vi "WiFi HttpUpload_Camera.vi"   [LabVIEW 2014]
doc: "This example shows how to take a picuture from ArduCAM mini 2MP camera and upload to HTTP server."
uses:
  PWS_ESP8266/PWS_ESP8266.lvlib
  QwaveSys_Interface/QwaveSys_Interface.lvlib
panel:
  # "Overview: Demonstrates how to use  HTTP upload function with AduCAM 2MP API to upload JPEG image to server. *ArduCAM required both SPI and I2C interface. (*I2C is for communication with PWS and SPI is for transfer image from FIFO buffer at high speed)\nRequirements: LabVIEW Full Development System,Arduino Compatible Compiler for LabVIEW,Programmable Wireless Stamp (PWS) Library.\nInstructions:\n1. Wire the ArduCAM to the Pmod SPI interface. refer below diagram.\n2. Wire the SCL,SDA from ArduCAM to the  I2C connector. refer below diagram. \n3. If this example has been loaded from the Arduino Compatible Compiler for LabVIEW, simply select Compile and Download.  Otherwise, open Tools>Arduino Compatible Compiler for LabVIEW in LabVIEW, then select File>Load VI, and select this VI and then Compile and Download.\n4. Open \"Serial Monitor\" by select \"Tools>Serial Monitor\" and select baud rate to 9600.\n5. Observe the data being print out on serial port monitor and RED led at USB TX LED will be blinking, by default at serial monitor it's will shown \"Event Connecting: (6) WL_DISCONNECTED\"\n6. Press and Hold FPROM_Btn for 2 sec or more to enter Smart Config mode. At serial monitor window its will shown \"Smart_Config_enter\"\n7. Using Smart Config Apps on Andriod/iOS to configure the WiFi network. refer getting start document for more information.\n8. After PWS has configured wifi network successfully. Observe  the \"Image Size: \" data being print out on serial port monitor. \n9. Goto \"http://iosys.link/pws/uploads/test.jpg\" to view the uploaded image file.\n\n#NOTE: \nArduCAM mini 2MP. The Arduino compatible based camera is a 2MP pixel camera sensor that supports output for raw RGB, RGB556/555, GRB422, YUV (422/420), YCbCr (4:2:2) and JPEG compression formats. This sensor is a great option for real time simple video applications.\nRefer: http://www.arducam.com/arducam-mini-released/"
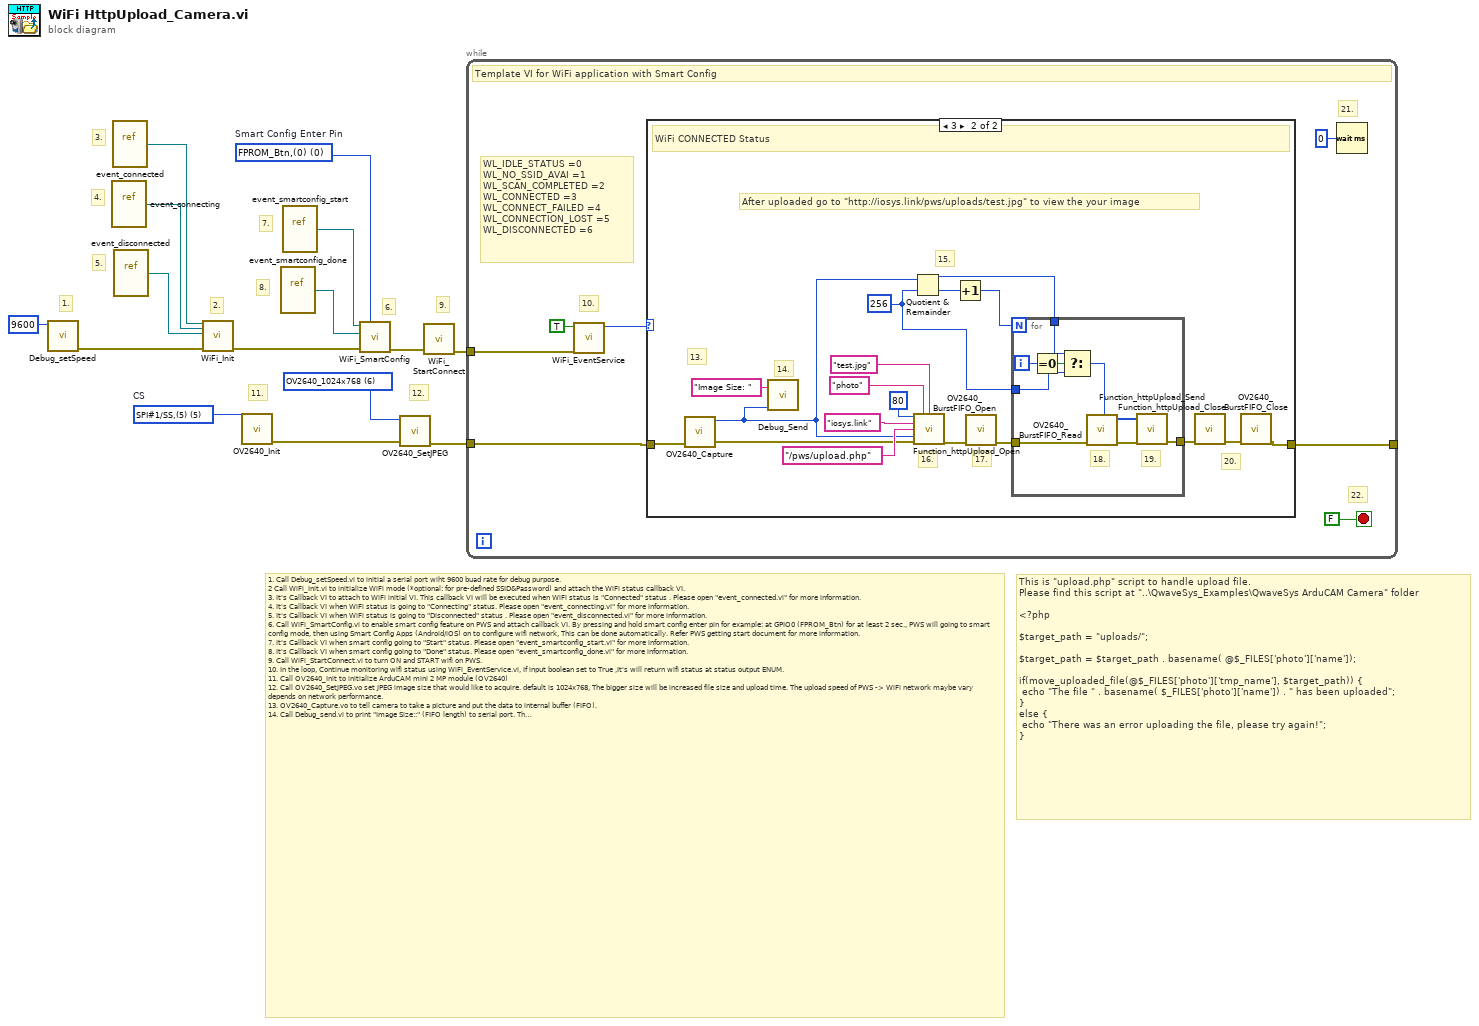
[diagram p0: block diagram]
diagram:
  w2 = u8 5 items=["SPI#1/SS,(5)"=5, "SPI#2/MOSI,(13)"=13, "SPI#3/MISO,(12)"=12, "SPI#4/SCLK,(14)"=14, "UART#1/CS,(15)"=15, "UART#2/TXD,(1)"=1, "UART#3/RXD,(3)"=3, "UART#4/LED,(16)"=16, "FPROM_Btn,(0)"=0, "SDCard_CS,(4)"=4, "I2C-SDA/TXD1,(2)"=2, "ADC0,(17)"=17]  # CS
  w4 = u16 6 items=["OV2640_160x120", "OV2640_176x144", "OV2640_320x240", "OV2640_352x288", "OV2640_640x480", "OV2640_800x600", "OV2640_1024x768", "OV2640_1280x1024", "OV2640_1600x1200"] ("resolution")
  w8 = u8 0 items=["SPI#1/SS,(5)"=5, "SPI#2/MOSI,(13)"=13, "SPI#3/MISO,(12)"=12, "SPI#4/SCLK,(14)"=14, "UART#1/CS,(15)"=15, "UART#2/TXD,(1)"=1, "UART#3/RXD,(3)"=3, "UART#4/LED,(16)"=16, "FPROM_Btn,(0)"=0, "SDCard_CS,(4)"=4, "I2C-SDA/TXD1,(2)"=2, "ADC0,(17)"=17]  # Smart Config Enter Pin
  # "This is \"upload.php\" script to handle upload file. \nPlease find this script at \"..\\QwaveSys_Examples\\QwaveSys ArduCAM Camera\" folder \n\n<?php\n\n$target_path = \"uploads/\";\n\n$target_path = $target_path . basename( @$_FILES['photo']['name']);\n\nif(move_uploaded_file(@$_FILES['photo']['tmp_name'], $target_path)) {\n\techo \"The file \" . basename( $_FILES['photo']['name']) . \" has been uploaded\";\n}\nelse {\n\techo \"There was an error uploading the file, please try again!\";\n}"
  # "12."
  # "11."
  # "9."
  # "8."
  # "7."
  # "1. Call Debug_setSpeed.vi to initial a serial port wiht 9600 buad rate for debug purpose.\n2 Call WiFi_Init.vi to initialize WiFi mode (*optional: for pre-defined SSID&Password) and attach the WiFi status callback VI.\n3. It's Callback VI to attach to WiFi initial VI. This callback VI will be executed when WiFi status is \"Connected\" status . Please open \"event_connected.vi\" for more information.\n4. It's Callback VI when WiFi status is going to \"Connecting\" status. Please open \"event_connecting.vi\" for more information.\n5. It's Callback VI when WiFi status is going to \"Disconnected\" status . Please open \"event_disconnected.vi\" for more information.\n6. Call WiFi_SmartConfig.vi to enable smart config feature on PWS and attach callback VI. By pressing and hold smart config enter pin for example: at GPIO0 (FPROM_Btn) for at least 2 sec., PWS will going to smart config mode, then using Smart Config Apps (Android/iOS) on to configure wifi network, This can be done automatically. Refer PWS getting start document for more information.\n7. It's Callback VI when smart config going to \"Start\" status. Please open \"event_smartconfig_start.vi\" for more information.\n8. It's Callback VI when smart config going to \"Done\" status. Please open \"event_smartconfig_done.vi\" for more information.\n9. Call WiFi_StartConnect.vi to turn ON and START wifi on PWS.\n10. In the loop, Continue monitoring wifi status using WiFi_EventService.vi, If input boolean set to True ,It's will return wifi status at status output ENUM. \n11. Call OV2640_Init to initialize ArduCAM mini 2 MP module (OV2640)\n12. Call OV2640_SetJPEG.vo set JPEG image size that would like to acquire. default is 1024x768, The bigger size will be increased file size and upload time. The upload speed of PWS -> WiFi network maybe vary depends on network performance.\n13. OV2640_Capture.vo to tell camera to take a picture and put the data to internal buffer (FIFO).\n14. Call Debug_send.vi to print \"Image Size::\" (FIFO length) to serial port. This is for debuging purpose.\n15.Calculate how many loop will be execute for upload, calc by using total file length/256 bytes, for split data for every 256 bytes.\n16. Call Function_httpUplaod_Open.vi to initialize uplaod function with required pararmetes (Hotst,URL,File Name)\n17. Call OV2640_BurstFIFO_Open.vi to tell the camera its ready to read data from FIFO buffer.\n18. In the for loop, Call OV2640_BurstFIFO_Read.vi to read image data from FIFO buffer for 256 bytes.\n19. In the for loop, Call Function_httpUplaod_Send.vi to start upload data to server for 256 bytes/loop.\n20. Closed reference for upload and camera functions.\n21. Delay 0 (ms) for each loop. As we need highest speed.\n22. Loop indefinitely.\n\n#NOTE: To view uploaded image file please go to \"\"http://iosys.link/pws/uploads/test.jpg\"\"\n\n\n\n\n\n2. Call MCP79410_init.vi to initialize onboard RTC chip (PWS is using Microchip MCP79410)\n3. Call RTC_GetDateTime.vi to read current date/time from RTC.\n4. Create 1D array of loop counter and random number to write to SD card.\n5. Call SD Data Logger.vi to write data to SD card with defined file name as \"PWSLog.csv\"\n6. Call Debug_send.vi to write Log Data to serial port. This is for debuging purpose.\n7. Delay 1 sec for every loop.\n8. Loop indefinitely.\n\n#NOTE: Error wire is used for flow control only and data on clusters cannot\nbe written nor accessed while deployed on an PWS target."
  # "6."
  # "5."
  # "4."
  # "3."
  # "2."
  # "1."
  n1 = call "Debug_setSpeed.vi"("Speed"=u32 9600) -> ("error out"=w12:errorcluster)  [unwired: 10 in]
  n2 = vi-ref "event_connecting.vi"() -> (w15:refnum<vi>)
  n3 = vi-ref "event_connected.vi"() -> (w14:refnum<vi>)
  n4 = vi-ref "event_disconnected.vi"() -> (w13:refnum<vi>)
  n5 = call "WiFi_Init.vi"("connected"=w14, "connecting"=w15, "disconnected"=w13, "error in (no error)"=w12) -> ("error out"=w7:errorcluster)  [unwired: 11 in]
  n6 = call "OV2640_Init.vi"("CS"=w2) -> ("error out"=w3:errorcluster)  [unwired: 9 in, 1 out]
  n7 = vi-ref "event_smartconfig_done.vi"() -> (w9:refnum<vi>)
  n8 = vi-ref "event_smartconfig_start.vi"() -> (w10:refnum<vi>)
  n9 = call "WiFi_SmartConfig.vi"("Smart Config Enter Pin"=w8, "error in (no error)"=w7, "smartconfig_done"=w9, "smartconfig_start"=w10) -> ("error out"=w6:errorcluster)  [unwired: 7 in]
  n10 = call "OV2640_SetJPEG.vi"("error in (no error)"=w3, "resolution"=w4) -> ("error out"=w1:errorcluster)  [unwired: 9 in]
  n11 = call "WiFi_StartConnect.vi"("error in (no error)"=w6) -> ("error out"=w5:errorcluster)  [unwired: 10 in]
  n12 = while {
    tunnel: [w19] -> _
    tunnel: w5 -> [w17]
    tunnel: w1 -> [w16]
    stop <- FALSE stop-if-true
    # "21."
    # "22."
    # "WL_IDLE_STATUS\t=0\nWL_NO_SSID_AVAI\t=1\nWL_SCAN_COMPLETED\t=2\nWL_CONNECTED\t=3\nWL_CONNECT_FAILED\t=4\nWL_CONNECTION_LOST\t=5\nWL_DISCONNECTED\t=6"
    # "10."
    # "Template VI for WiFi application with Smart Config"
    n13 = call "WiFi_EventService.vi"("error in (no error)"=w17, "wait for connected (True)"=TRUE) -> ("Status"=w20:u16)  [unwired: 8 in, 1 out]
    n14 = case shown="3" w20 {
      tunnel: w16 -> [w23 w26]
      tunnel: [w23 w24] -> w19
      frame 0, Default {
        # "12."
        # "Default Case: Using for handle IDLE or DISCONNECTED status"
      }
      frame 3 {
        w30 = u32 256 ("y")
        # "After uploaded go to \"http://iosys.link/pws/uploads/test.jpg\" to view the your image"
        # "20."
        # "17."
        # "16."
        # "15."
        # "14."
        # "13."
        # "WiFi CONNECTED Status"
        n15 = call "OV2640_Capture.vi"("error in (no error)"=w26) -> ("error out"=w25:errorcluster, "FIFO Length"=w28:u32)  [unwired: 9 in]
        n16 = call "Debug_Send.vi"("Name"="Image Size: ", "DATA"=w28) -> ()  [unwired: 10 in]
        n17 = Quotient & Remainder(x=w28, y=w30) -> (x-y*floor(x/y)=w31:u32, floor(x/y)=w35:u32)
        n18 = call "Function_httpUpload_Open.vi"("Port"=i8 80, "Name"="photo", "Filename"="test.jpg", "Host"="iosys.link", "URI"="/pws/upload.php", "Upload Lenght"=w28, "error in (no error)"=w25) -> ("error out"=w37:errorcluster)  [unwired: 8 in]
        n19 = Increment(x=w35) -> (x+1=w32:u32)
        n20 = call "OV2640_BurstFIFO_Open.vi"("error in (no error)"=w37) -> ("error out"=w34:errorcluster)  [unwired: 10 in]
        n21 = for {
          N: w32 -> [_]
          tunnel: w34 -> [w48]
          tunnel: [w47] -> w33
          tunnel: w31 -> [w44]
          tunnel: w30 -> [w43]
          i -> [w46]
          # "19."
          # "18."
          n22 = Equal To 0?(x=w46) -> (x = 0?=w45:bool)
          n23 = Select(t=w44, s=w45, f=w43) -> (s? t:f=w42:u32)
          n24 = call "OV2640_BurstFIFO_Read.vi"("error in (no error)"=w48, "Lenght"=w42) -> ("error out"=w50:errorcluster, "DATA"=w49:u8[])  [unwired: 8 in]
          n25 = call "Function_httpUpload_Send.vi"("error in (no error)"=w50, "DATA"=w49) -> ("error out"=w47:errorcluster)  [unwired: 9 in]
        }
        n26 = call "Function_httpUpload_Close.vi"("error in (no error)"=w33) -> ("error out"=w36:errorcluster)  [unwired: 10 in]
        n27 = call "OV2640_BurstFIFO_Close.vi"("error in (no error)"=w36) -> ("error out"=w24:errorcluster)  [unwired: 10 in]
      }
    }
    n28 = Wait (ms)(milliseconds to wait=u32 0) -> ()  [unwired: 1 out]
  }
